vi "Config Reader.vi"(0 "Path":path, 5 "error in (no error)":errorcluster) -> (1 "Withdraw rate":dbl=2.0, 2 "Withdraw \nVolume unit":u16(ring) items=["µL", "nL", "mL"], 4 "Withdraw \nVolume":i32=100, 6 "Default Current Force":i32=30 min=0 max=100 step=1, 7 "Default Volume unit":u16(ring) items=["µL", "nL", "mL"], 8 "Mode":string, 9 "Withdraw Rate \nUnits":u32(ring)=3 items=["ml/hr", "ml/min", "ul/hr", "ul/min", "ul/sec", "nl/sec"], 11 "Default Syringe Volume Unit":u16(ring) items=["µL", "nL", "mL"], 12 "Default Flow Rate Units (1:ml/min)":u32(ring)=3 items=["ml/hr", "ml/min", "ul/hr", "ul/min", "ul/sec", "nl/sec"], 13 "Default Volume":i32=100, 14 "VISA Refnum out":refnum<visa-resource-name>, 15 "Default Infusion rate":dbl=2.0, 17 "Default Syringe Volume":i32=30 min=0 max=100 step=1, 18 "Default Syringe Diameter (mm)":dbl=4.86 min=0.01 max=49.99 step=0.01 format="%.2g", 19 "error out":errorcluster)   [LabVIEW 2016]
uses:
  <vilib>/Utility/config.llb/Read Key (String).vi
  <vilib>/Utility/config.llb/Read Key (Double).vi
  <vilib>/Utility/config.llb/Read Key (I32).vi
  <vilib>/Utility/config.llb/NI_LVConfig.lvlib
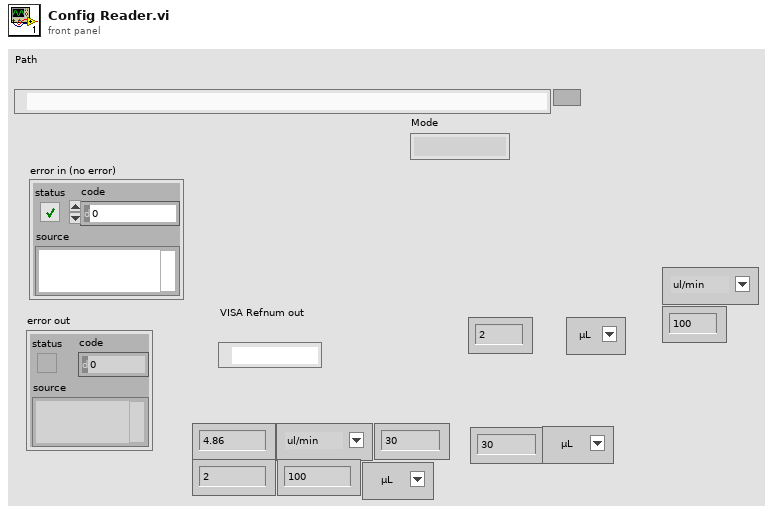
[diagram p1: front panel]
types:
  T1 = cluster{"Vendor ID":string, "Product ID":string, "S/N":string}
  T2 = typedef "NI_LVConfig.lvlib/Config Data RefNum.ctl" = refnum<k1>
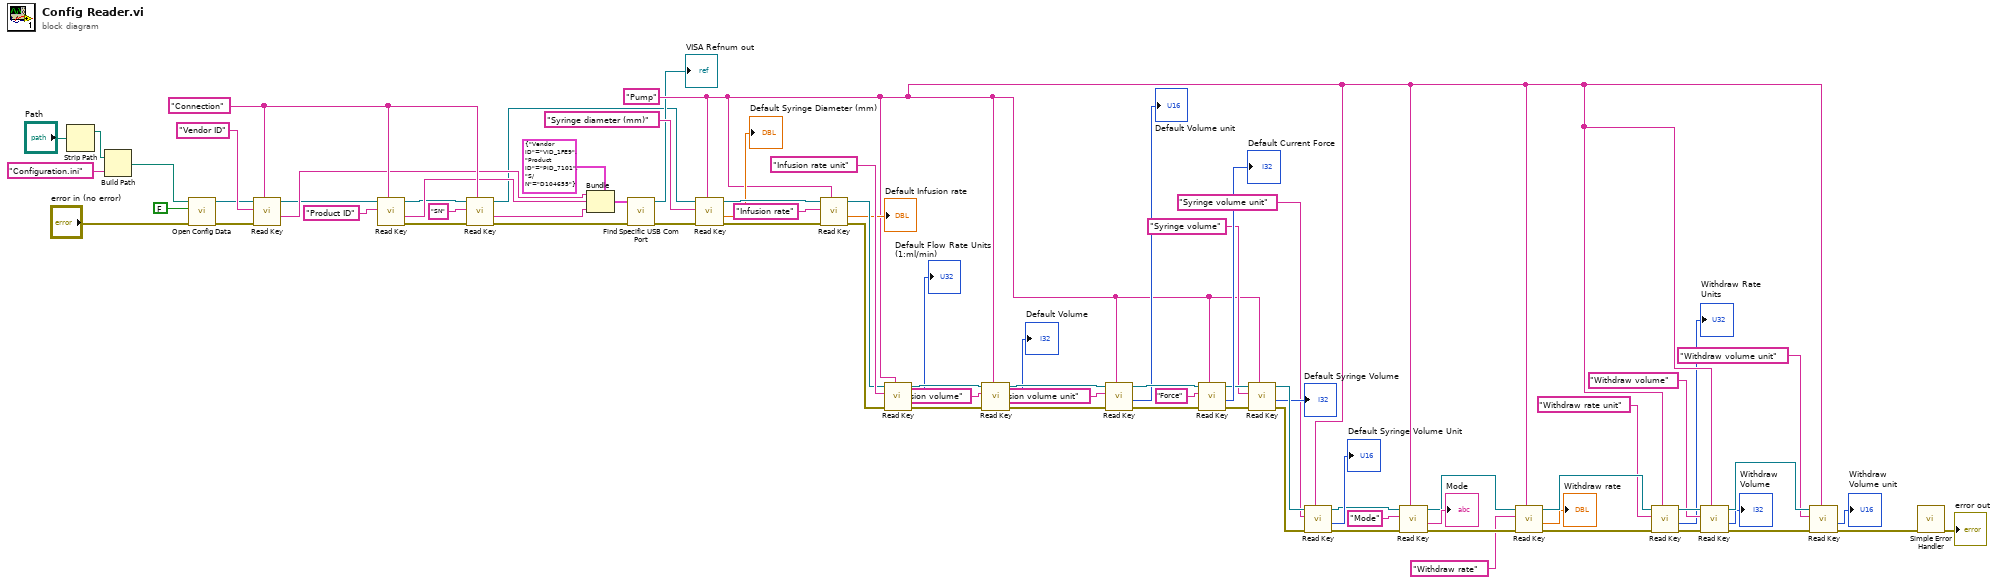
[diagram p0: block diagram]
diagram:
  w24 = "Pump" ("section")
  w14 = "Connection" ("section")
  n1 = Strip Path(path="Path") -> (stripped path=w58:path)  [unwired: 1 out]
  n2 = Build Path(base path=w58, name or relative path="Configuration.ini") -> (appended path=w56:path)
  n3 = call <vilib>:"Open Config Data.vi"("error in (no error)"="error in (no error)", "create file if necessary (T)"=FALSE, "configuration file path"=w56) -> ("error out"=w71:errorcluster, "refnum"=w60:T2)  [unwired: 6 in, 1 out]
  n4 = call-poly <vilib>:"Read Key.vi"("section"=w14, "error in (no error)"=w71, "key"="Vendor ID", "refnum"=w60) -> ("value"=w10:string, "refnum out"=w6:T2)  [unwired: 4 in, 2 out]
  n5 = call-poly <vilib>:"Read Key.vi"("section"=w14, "key"="Product ID", "refnum"=w6) -> ("error out"=w7:errorcluster, "value"=w9:string, "refnum out"=w5:T2)  [unwired: 5 in, 1 out]
  n6 = call-poly <vilib>:"Read Key.vi"("section"=w14, "error in (no error)"=w7, "key"="SN", "refnum"=w5) -> ("error out"=w2:errorcluster, "value"=w8:string, "refnum out"=w4:T2)  [unwired: 4 in, 1 out]
  n7 = Bundle(cluster=T1 {"Vendor ID"="VID_1FE9", "Product ID"="PID_7101", "S/N"="D104655"} ("Identifiers (regular expressions)"), "Vendor ID"=w10, "Product ID"=w9, "S/N"=w8) -> (w3:T1)
  n8 = call "Find Specific USB Com Port.vi"("Error In"=w2, "Identifiers (regular expressions)"=w3) -> ("Error Out"=w1:errorcluster, "Com Port"=→"VISA Refnum out":refnum<visa-resource-name>)  [unwired: 3 in, 1 out]
  n9 = call-poly <vilib>:"Read Key.vi"("section"=w24, "error in (no error)"=w1, "key"="Syringe diameter (mm)", "refnum"=w4) -> ("error out"=w72:errorcluster, "value"=→"Default Syringe Diameter (mm)":dbl, "refnum out"=w62:T2)  [unwired: 4 in, 1 out]
  n10 = call-poly <vilib>:"Read Key.vi"("section"=w24, "error in (no error)"=w72, "key"="Infusion rate", "refnum"=w62) -> ("error out"=w73:errorcluster, "value"=→"Default Infusion rate":dbl, "refnum out"=w63:T2)  [unwired: 4 in, 1 out]
  n11 = call-poly <vilib>:"Read Key.vi"("section"=w24, "error in (no error)"=w73, "key"="Infusion rate unit", "refnum"=w63) -> ("error out"=w74:errorcluster, "value"=→"Default Flow Rate Units (1:ml/min)":i32, "refnum out"=w64:T2)  [unwired: 4 in, 1 out]
  n12 = call-poly <vilib>:"Read Key.vi"("section"=w24, "error in (no error)"=w74, "key"="Infusion volume", "refnum"=w64) -> ("error out"=w75:errorcluster, "value"=→"Default Volume":i32, "refnum out"=w65:T2)  [unwired: 4 in, 1 out]
  n13 = call-poly <vilib>:"Read Key.vi"("section"=w24, "error in (no error)"=w75, "key"="Infusion volume unit", "refnum"=w65) -> ("error out"=w54:errorcluster, "value"=→"Default Volume unit":i32, "refnum out"=w76:T2)  [unwired: 4 in, 1 out]
  n14 = call-poly <vilib>:"Read Key.vi"("section"=w24, "error in (no error)"=w54, "key"="Force", "refnum"=w76) -> ("error out"=w45:errorcluster, "value"=→"Default Current Force":i32, "refnum out"=w44:T2)  [unwired: 4 in, 1 out]
  n15 = call-poly <vilib>:"Read Key.vi"("section"=w24, "error in (no error)"=w45, "key"="Syringe volume", "refnum"=w44) -> ("error out"=w42:errorcluster, "value"=→"Default Syringe Volume":i32, "refnum out"=w43:T2)  [unwired: 4 in, 1 out]
  n16 = call-poly <vilib>:"Read Key.vi"("section"=w24, "error in (no error)"=w42, "key"="Syringe volume unit", "refnum"=w43) -> ("error out"=w37:errorcluster, "value"=→"Default Syringe Volume Unit":i32, "refnum out"=w34:T2)  [unwired: 4 in, 1 out]
  n17 = call-poly <vilib>:"Read Key.vi"("section"=w24, "error in (no error)"=w37, "key"="Mode", "refnum"=w34) -> ("error out"=w25:errorcluster, "value"=→"Mode":string, "refnum out"=w33:T2)  [unwired: 4 in, 1 out]
  n18 = call-poly <vilib>:"Read Key.vi"("section"=w24, "error in (no error)"=w25, "key"="Withdraw rate", "refnum"=w33) -> ("error out"=w26:errorcluster, "value"=→"Withdraw rate":dbl, "refnum out"=w32:T2)  [unwired: 4 in, 1 out]
  n19 = call-poly <vilib>:"Read Key.vi"("section"=w24, "error in (no error)"=w26, "key"="Withdraw rate unit", "refnum"=w32) -> ("error out"=w27:errorcluster, "value"=→"Withdraw Rate \nUnits":i32, "refnum out"=w31:T2)  [unwired: 4 in, 1 out]
  n20 = call-poly <vilib>:"Read Key.vi"("section"=w24, "error in (no error)"=w27, "key"="Withdraw volume", "refnum"=w31) -> ("error out"=w28:errorcluster, "value"=→"Withdraw \nVolume":i32, "refnum out"=w30:T2)  [unwired: 4 in, 1 out]
  n21 = call-poly <vilib>:"Read Key.vi"("section"=w24, "error in (no error)"=w28, "key"="Withdraw volume unit", "refnum"=w30) -> ("error out"=w29:errorcluster, "value"=→"Withdraw \nVolume unit":i32)  [unwired: 4 in, 2 out]
  n22 = call <vilib>:"Simple Error Handler.vi"("error in (no error)"=w29) -> ("error out"=→"error out":errorcluster)  [unwired: 4 in, 4 out]
